vi "Get 1D String.vi"(5 "format string (%s)":string="%s", 7 "key description":string, 8 "sections":string[](array[string]), 9 "string":string[](array[string]), 11 "info data":string) -> (0 "sections out":string[](array[string]), 2 "value":string[](array[string]), 3 "info data out":string)   [LabVIEW 2013, in "infolib.lvlib"]
doc: "Reads horizontal or vertical vector of strings. If section is entered it searches the key in the section(s)."
uses:
  infolib.lvlib
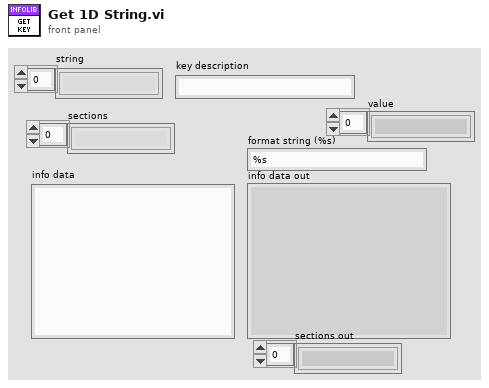
[diagram p1: front panel]
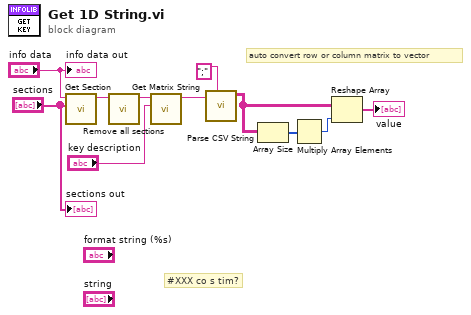
[diagram p0: block diagram]
diagram:
  # "#XXX co s tim?"
  # "auto convert row or column matrix to vector"
  n1 = call "Get Section.vi"("sections"="sections", "info data"="info data") -> ("section part"=w11:string)  [unwired: 8 in, 1 out]
  n2 = call "Remove all sections.vi"("info data"=w11) -> ("info data out"=w8:string)  [unwired: 10 in]
  n3 = call "Get Matrix String.vi"("matrix key"="key description", "info data"=w8) -> ("matrix part"=w3:string)  [unwired: 8 in, 1 out]
  n4 = call "Parse CSV String.vi"("delimiter (,)"=";" ("delimiter (Tab)"), "CSV string"=w3) -> ("2-D array"=w1:string[][])  [unwired: 8 in, 1 out]
  n5 = Array Size(array=w1) -> (size(s)=w6:i32[])
  n6 = Multiply Array Elements(1:w6) -> (0:w5:i32)
  n7 = Reshape Array(w1, w5) -> (→"value":string[])
  "info data out" <- "info data"
  "sections out" <- "sections"
